vi "test Broadcast Function Code Typedef.vi"(11 "Test Case In":refnum<class "Function Code Typedef Test.lvclass">) -> (0 "error out":errorcluster, 3 "Test Case Out":refnum<class "Function Code Typedef Test.lvclass">)   [LabVIEW 2024, in "Function Code Typedef Test.lvclass"]
uses:
  Function Code Typedef Test.lvclass
  C:/Program Files/National Instruments/LabVIEW 2024/vi.lib/Astemes/LUnit/Test Case.lvclass
  <vilib>/Astemes/LUnit/Test Case.lvclass/Test Case.ctl
  4993e8ee-a06a-463a-9684-69129f64d5ce.vi
  <vilib>/Astemes/LUnit/Append Pass Result.vi
  <vilib>/Astemes/LUnit/Append Fail Result.vi
  <vilib>/Astemes/LUnit/Describe Comparison.vi
  4993e8ee-a06a-463a-9684-69129f64d5ce.vi/9c5d11cd-9439-4240-a1ee-d9baace9c924.vi
  <vilib>/Astemes/LUnit/Run In UI.vi
  <vilib>/Utility/error.llb/Clear Errors.vi
  <vilib>/Astemes/LUnit/Describe Variant.vi
  Function Code Typedef Test.lvclass/Function Code Typedef Test.ctl
  CANopen/Broadcast Function Code.ctl
  CANopen/CANopen.lvclass
panel:
  out "x = y?":bool
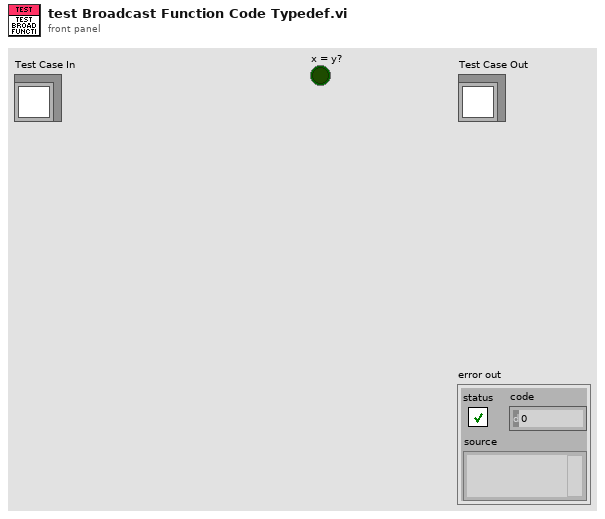
[diagram p1: front panel]
types:
  T1 = typedef "CANopen.lvlib/CANopen.lvclass/Broadcast Function Code.ctl" = map{string, i32}
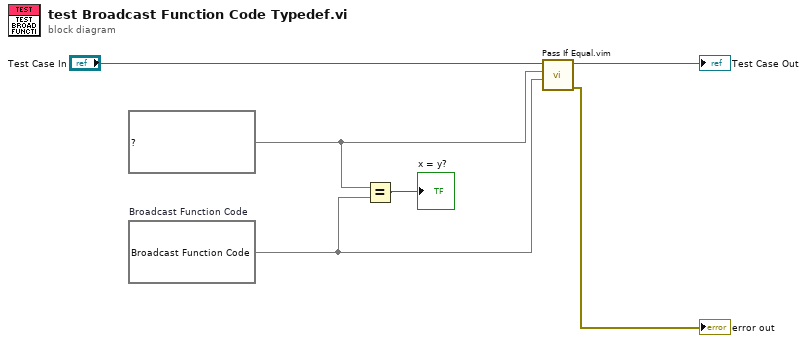
[diagram p0: block diagram]
diagram:
  w3 = map{string, i32} {"NMT"=0, "SYNC"=1, "TIME"=2} ("Function Code")
  w2 = T1 {"NMT"=0, "SYNC"=1, "TIME"=2}  # Broadcast Function Code
  n1 = Equal?(x=w3, y=w2) -> (x = y?=→"x = y?":bool)
  n2 = call "Pass If Equal.vim"("Actual"=w2, "Expected"=w3, "LUnit Test Case In"="Test Case In") -> ("error out"=→"error out":errorcluster, "LUnit Test Case Out"=→"Test Case Out":refnum<class "Function Code Typedef Test.lvclass">)  [unwired: 7 in]
